vi "logger.vi"(0 "Name":string, 5 "ID":string, 7 "Pin":string, 9 "User/Admin":string, 11 "Success?":string) -> ()   [LabVIEW 2019]
uses:
  <vilib>/Utility/file.llb/Write Delimited Spreadsheet (string).vi
panel:
  out "String":string
  out "appended array":string[](array[string])
  out "time string":string
  out "date string":string
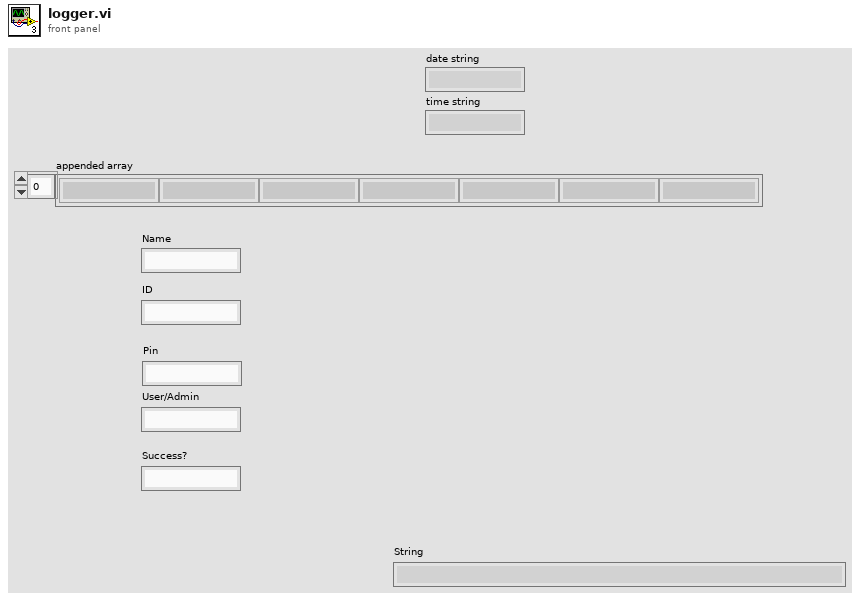
[diagram p1: front panel]
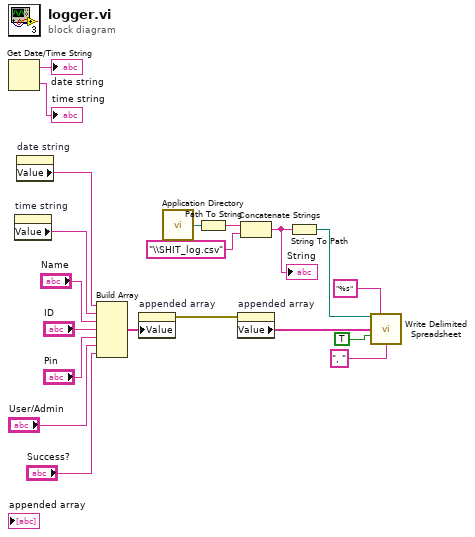
[diagram p0: block diagram]
diagram:
  n1 = Get Date/Time String() -> (date string=→"date string":string, time string=→"time string":string)  [unwired: 3 in]
  n2 = property on="time string" class="Str"() -> ("Value"=w17:string)  [unwired: 2 in, 2 out]
  n3 = property on="date string" class="Str"() -> ("Value"=w18:string)  [unwired: 2 in, 2 out]
  n4 = Build Array(w18, w17, "Name", "ID", "Pin", "User/Admin", "Success?") -> (w2:string[])
  n5 = property on="appended array" class="Arr (strict)"("Value"=w2) -> (error out=w1:errorcluster)  [unwired: 2 in, 1 out]
  n6 = call <vilib>:"Application Directory.vi"() -> ("Application Directory"=w8:path)
  n7 = Path To String(path=w8) -> (string=w7:string)
  n8 = property on="appended array" class="Arr (strict)"(error in=w1) -> ("Value"=w11:string[])  [unwired: 1 in, 2 out]
  n9 = Concatenate Strings(w7, "\\SHIT_log.csv" ("search string")) -> (w4:string)
  "String" <- w4
  n10 = String To Path(string=w4) -> (path=w5:path)
  n11 = call-poly <vilib>:"Write Delimited Spreadsheet.vi"("file path (dialog if empty)"=w5, "format (%s)"="%s", "1D data"=w11, "append to file? (new file:F)"=TRUE, "delimiter (\\t)"=", " ("delimiter (\\t)")) -> ()  [unwired: 9 in, 2 out]
